vi "CAN_Send_And_Receive_AP_Data_3.vi"(7 "File Path":path, 8 "Current Position In":i16 format="%02x", 9 "AP DataIn":i16[][](array[numeric]) format="%02x", 10 "AP Data Type":T1, 11 "NetworkObjHandle":T2) -> (0 "Current Position":i16 format="%02x", 2 "AP Data":i16[][](array[numeric]) format="%02x")   [LabVIEW 2012]
uses:
  <vilib>/nican/nican.llb/xobjhandle.ctl
  <userlib>/type defs/17x AP Data Type.ctl
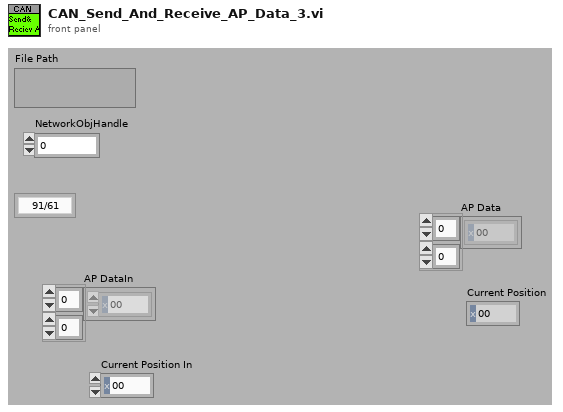
[diagram p1: front panel]
types:
  T1 = typedef "17x AP Data Type.ctl" = enum16{"91/61", "92/62", "93/63", "67", "68", "6F", "71"}
  T2 = typedef "xobjhandle.ctl" = u32
  T3 = cluster{"File Path":path, "NetworkObjHandle":T2, "Rx Msg":u8[][], "TxRx Data":string[][]}
  T4 = typedef "CanFrameTimed.ctl" = cluster{"Timestamp":dbl, "ArbitrationId":u32, "IsRemote":u8, "DataLength":u8, "Data":u8[]}
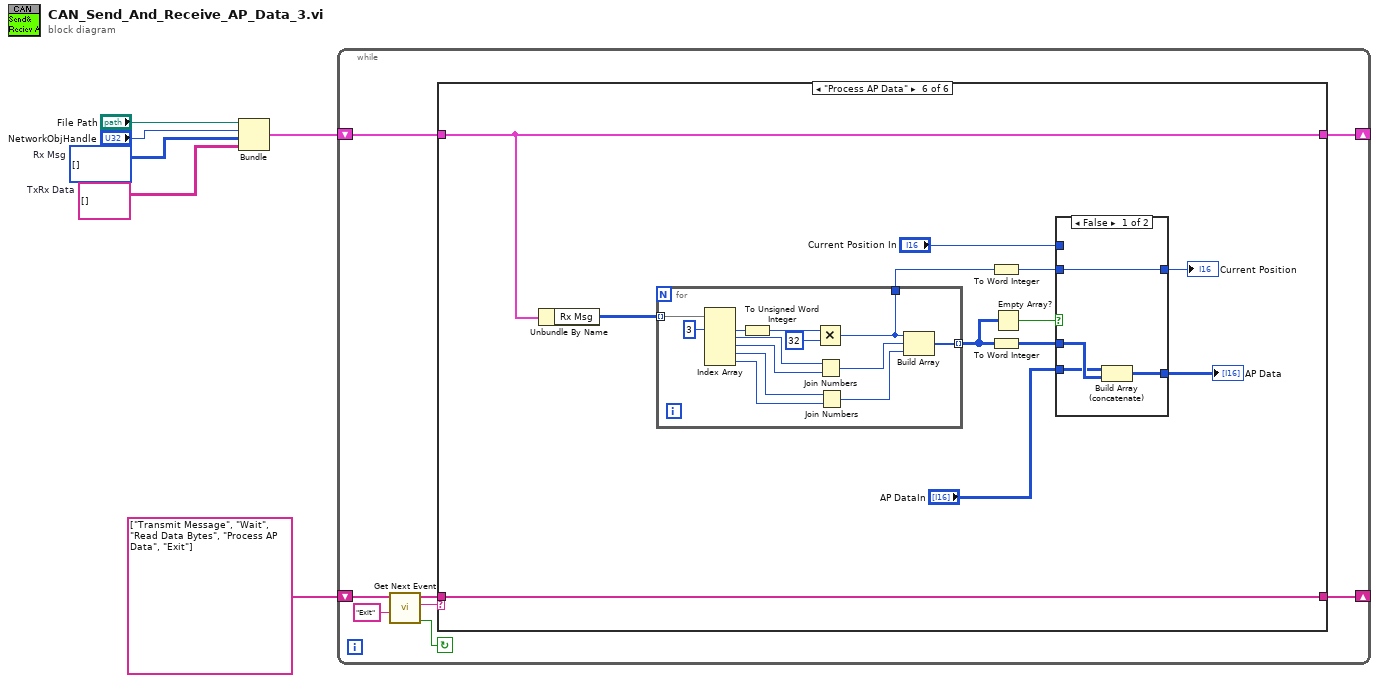
[diagram p0: block diagram]
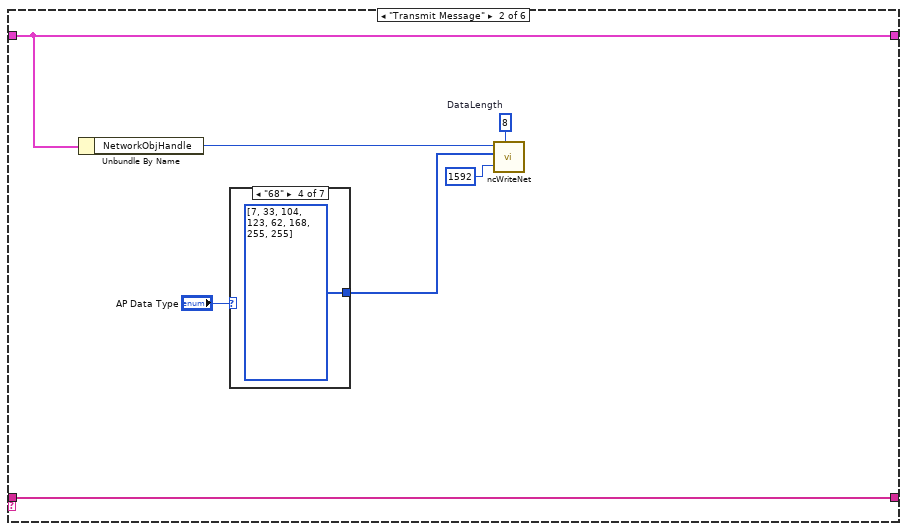
[diagram p3: hidden frame]
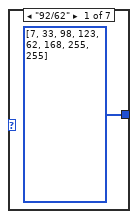
[diagram p4: hidden frame]
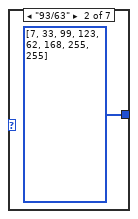
[diagram p5: hidden frame]
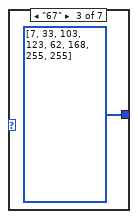
[diagram p6: hidden frame]
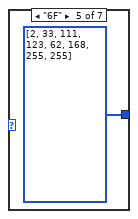
[diagram p7: hidden frame]
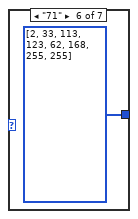
[diagram p8: hidden frame]
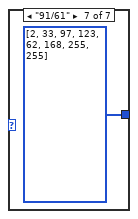
[diagram p9: hidden frame]
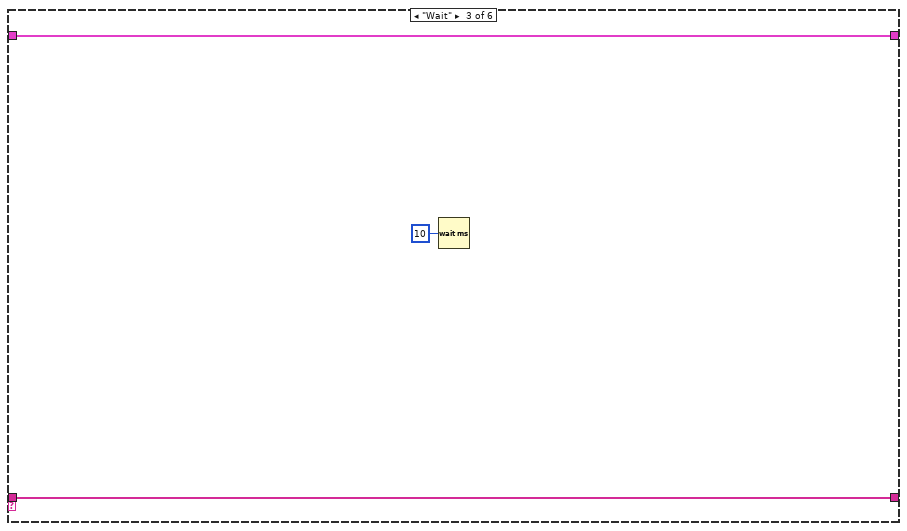
[diagram p10: hidden frame]
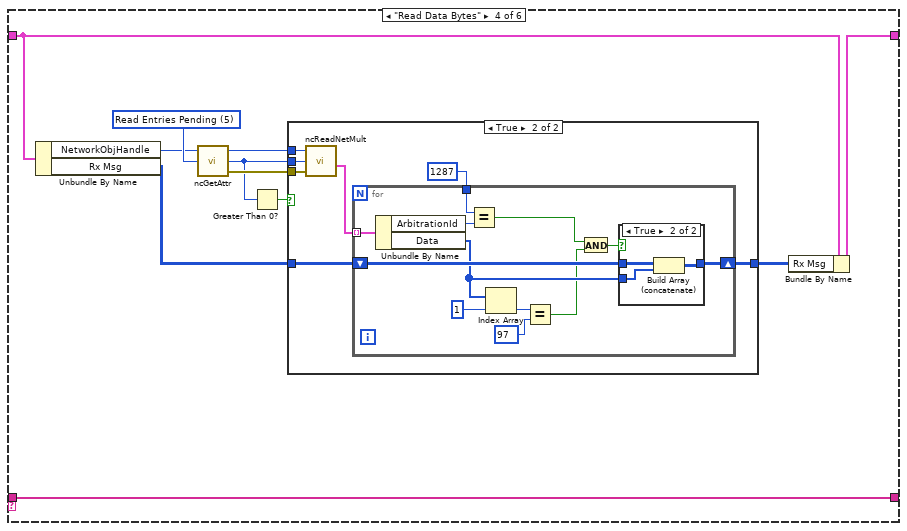
[diagram p11: hidden frame]
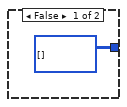
[diagram p12: hidden frame]
diagram:
  w2 = string[][] []  # TxRx Data
  w4 = u8[][] []  # Rx Msg
  n1 = Bundle("File Path"="File Path", "NetworkObjHandle"="NetworkObjHandle", "Rx Msg"=w4, "TxRx Data"=w2) -> (w5:T3)  [unwired: 1 in]
  n2 = while {
    shift-right: [w11] -> _
    shift-left: string[] ["Transmit Message", "Wait", "Read Data Bytes", "Process AP Data", "Exit"] ("event queue out") -> [w10]
    shift-right: [w8] -> _
    shift-left: w5 -> [w9]
    stop <- w14 continue-if-true
    n3 = call <userlib>:"Get Next Event.vi"("Exit Event"="Exit", "event queue in"=w10) -> ("Condition (Exit:F)"=w14:bool, "next event"=w13:string, "event queue out"=w12:string[])  [unwired: 3 in]
    n4 = case shown="\"Process AP Data\"" w13 {
      tunnel: w12 -> [w16 w17 w31 w35 w70 w82]
      tunnel: [w16 w17 w31 w35 w70 w82] -> w11
      tunnel: w9 -> [w15 w20 w32 w39 w69 w81]
      tunnel: [w15 w20 w32 w38 w69 w81] -> w8
      frame "Error", Default {
      }
      frame "Transmit Message" {
        w22 = u32 8  # DataLength
        n5 = Unbundle By Name(w20) -> ("NetworkObjHandle"=w23:T2)
        n6 = case shown="\"68\"" "AP Data Type" {
          tunnel: [u8[] [7, 33, 98, 123, 62, 168, 255, 255] ("Tx Msg") u8[] [7, 33, 99, 123, 62, 168, 255, 255] ("Tx Msg") u8[] [7, 33, 103, 123, 62, 168, 255, 255] ("Tx Msg") u8[] [7, 33, 104, 123, 62, 168, 255, 255] ("Tx Msg") u8[] [2, 33, 111, 123, 62, 168, 255, 255] ("Tx Msg") u8[] [2, 33, 113, 123, 62, 168, 255, 255] ("Tx Msg") u8[] [2, 33, 97, 123, 62, 168, 255, 255] ("Tx Msg")] -> w18
          frame "92/62" {
          }
          frame "93/63" {
          }
          frame "67" {
          }
          frame "68" {
          }
          frame "6F" {
          }
          frame "71" {
          }
          frame "91/61" {
          }
        }
        n7 = call <vilib>:"ncWriteNet.vi"("ArbitrationId"=u32 1592 ("Tx Arbitration Id"), "DataLength"=w22, "Data"=w18, "ObjHandle in"=w23) -> ()  [unwired: 2 in, 2 out]
      }
      frame "Wait" {
        n8 = Wait (ms)(milliseconds to wait=u32 10) -> ()  [unwired: 1 out]
      }
      frame "Read Data Bytes" {
        w42 = u32 5 items=["(reserved)", "Protocol Version", "Software Version", "Object State", "(reserved)", "Read Entries Pending", "Write Entries Pending", "ReadMult Size for Notification", "Listen Only?", "Self Reception?", "Transmit Error Counter", "Receive Error Counter", "Single Shot Transmit?", "Series 2 Filter Mode", "Series 2 Mask", "Series 2 Comparator", "Serial Number", "Form Factor", "Series", "Transceiver Type", "Interface Number", "Series 2 Error/Arb Capture", "Transceiver Mode", "Transceiver External Outputs", "Transceiver External Inputs", "Start Trigger Behavior", "Log Comm Warnings", "User RTSI Frame", "Transmit Mode", "Log Start Trigger?", "Timestamp Format", "Master Timebase Rate", "Virtual Bus Timing"] ("AttrId")
        n9 = Unbundle By Name(w39) -> ("NetworkObjHandle"=w36:T2, "Rx Msg"=w34:u8[][])
        n10 = call <vilib>:"ncGetAttr.vi"("AttrId"=w42, "ObjHandle in"=w36) -> ("Error out"=w44:errorcluster, "AttrValue"=w40:u32, "ObjHandle out"=w43:T2)  [unwired: 1 in]
        n11 = Greater Than 0?(x=w40) -> (x > 0?=w41:bool)
        n12 = case shown="True" w41 {
          tunnel: w40 -> [_ w52]
          tunnel: w44 -> [_ w51]
          tunnel: w43 -> [_ w50]
          tunnel: [u8[][] [] ("Data Array") w48] -> w37
          tunnel: w34 -> [_ w47]
          frame False {
          }
          frame True {
            n13 = call <vilib>:"ncReadNetMult.vi"("ObjHandle in"=w50, "Requested Number of Frames"=w52, "Error in"=w51) -> ("Data"=w49:T4[])  [unwired: 3 out]
            n14 = for {
              tunnel: w49 -> [w64] mode=indexing
              shift-right: [w62] -> w48
              shift-left: w47 -> [w61]
              tunnel: u32 1287 ("Tx Arbitration Id") -> [w55]
              n15 = Unbundle By Name(w64) -> ("ArbitrationId"=w63:u32, "Data"=w59:u8[])
              n16 = Equal?(x=w55, y=w63) -> (x = y?=w58:bool)
              n17 = Index Array(array=w59, index=1) -> (element=w57:u8)
              n18 = Equal?(x=w57, y=u8 97 ("Numeric")) -> (x = y?=w56:bool)
              n19 = And(x=w58, y=w56) -> (x .and. y?=w60:bool)
              n20 = case shown="True" w60 {
                tunnel: w59 -> [_ w67]
                tunnel: [w65 w66] -> w62
                tunnel: w61 -> [w65 w68]
                frame False {
                }
                frame True {
                  n21 = Build Array (concatenate)(w68, w67) -> (w66:u8[][])
                }
              }
            }
          }
        }
        n22 = Bundle By Name(cluster=w39, "Rx Msg"=w37) -> (w38:T3)
      }
      frame "Exit" {
      }
      frame "Process AP Data" {
        n23 = Unbundle By Name(w81) -> ("Rx Msg"=w80:u8[][])
        n24 = for {
          tunnel: w80 -> [w101] mode=indexing
          tunnel: [w91] -> w78 mode=indexing
          tunnel: [w89] -> w74
          n25 = Index Array(array=w101, index #1=3 ("index")) -> (element #1=w99:u8, element #2=w97:u8, element #3=w96:u8, element #4=w95:u8, element #5=w94:u8)  [unwired: 4 in]
          n26 = To Unsigned Word Integer(number=w99) -> (unsigned 16bit integer=w90:u16)
          n27 = Multiply(x=w90, y=u16 32) -> (x*y=w89:u16)
          n28 = Join Numbers(hi=w97, lo=w96) -> ((hi.lo)=w93:u16)
          n29 = Join Numbers(hi=w95, lo=w94) -> ((hi.lo)=w92:u16)
          n30 = Build Array(w89, w93, w92) -> (w91:u16[])
        }
        n31 = To Word Integer(number=w74) -> (16bit integer=w72:i16)
        n32 = To Word Integer(number=w78) -> (16bit integer=w71:i16[][])
        n33 = Empty Array?(array=w78) -> (empty?=w79:bool)
        n34 = case shown="False" w79 {
          tunnel: [w86 w88] -> w76
          tunnel: w71 -> [w85 _]
          tunnel: "AP DataIn" -> [w84 w88]
          tunnel: w72 -> [w83 _]
          tunnel: [w83 w87] -> w73
          tunnel: "Current Position In" -> [_ w87]
          frame False {
            n35 = Build Array (concatenate)(w84, w85) -> (w86:i16[][])
          }
          frame True {
          }
        }
        "AP Data" <- w76
        "Current Position" <- w73
      }
    }
  }
